vi "Scan Barcode enqueue.vi"(5 "Enum Selection":T2, 6 "Enqueue N":T1[](array[typedef]), 7 "Error In":errorcluster, 9 "Enqueue":T1, 10 "queue in":refnum<queue>) -> (0 "error out":errorcluster, 2 "D-enqueue":T1, 3 "queue Out":refnum<queue>)   [LabVIEW 2015]
uses:
  Test selectionSB.ctl
  Test seqSB.ctl
panel:
  out "Denueue N":T1[](array[typedef])
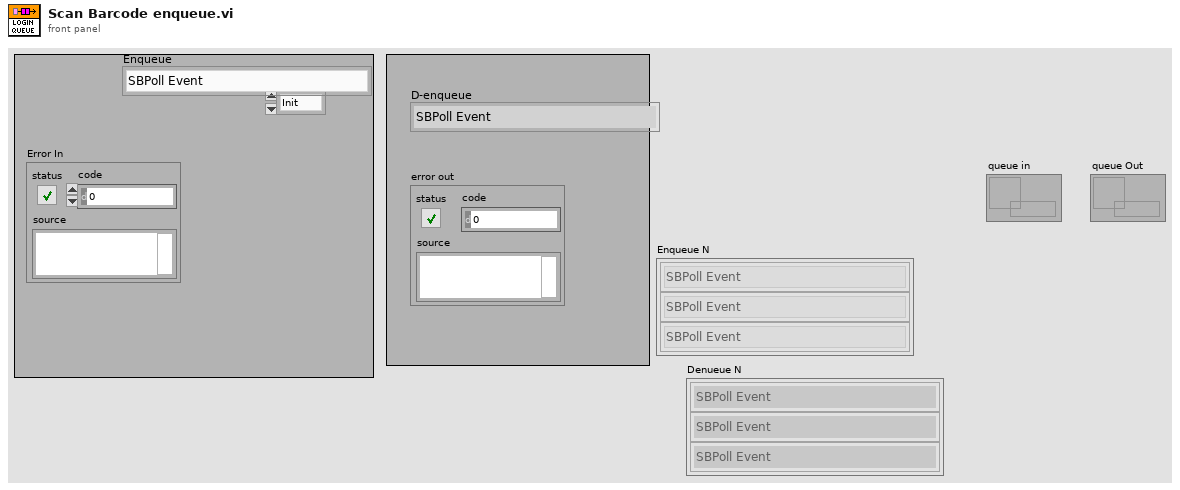
[diagram p1: front panel]
types:
  T1 = typedef "Test seqSB.ctl" = enum16{"SBPoll Event", "SBinitialize", "SB Comport Check1", "SB Comport Check2", "SB Comport Check3", "SB Comport Check4", "SB Exit"}
  T2 = typedef "Test selectionSB.ctl" = enum16{"Init", "Enqueue ", "Enqueue N", "Enqueue in stack", "Enqueue in stack N", "Dequeue", "Dequeue N", "Flush", "Release Queue"}
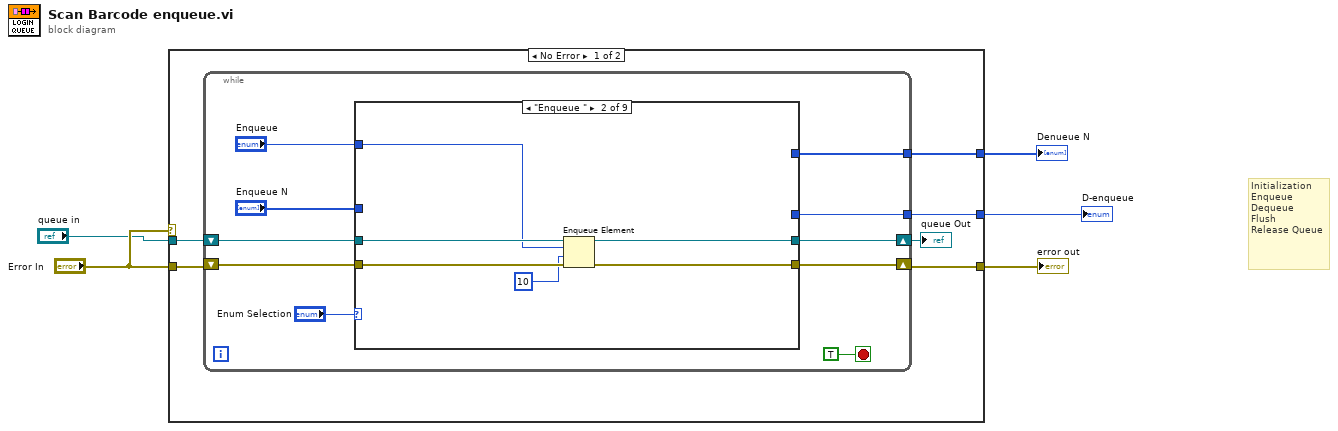
[diagram p0: block diagram]
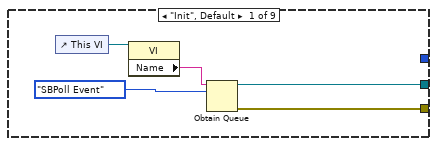
[diagram p2: hidden frame]
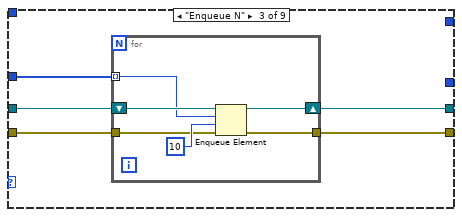
[diagram p3: hidden frame]
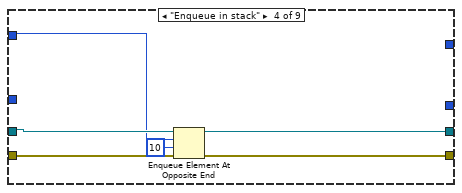
[diagram p4: hidden frame]
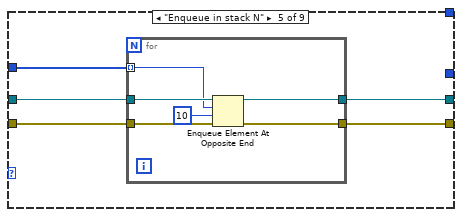
[diagram p5: hidden frame]
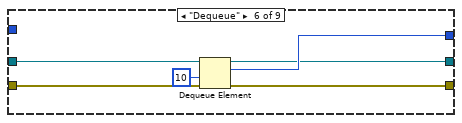
[diagram p6: hidden frame]
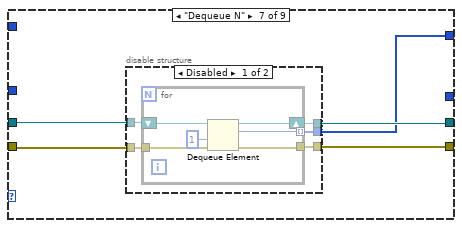
[diagram p7: hidden frame]
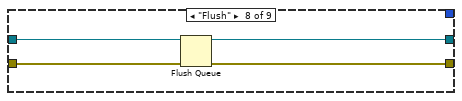
[diagram p9: hidden frame]
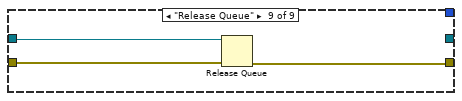
[diagram p10: hidden frame]
diagram:
  # "Initialization\nEnqueue\nDequeue\nFlush\nRelease Queue"
  n1 = case shown="No Error" "Error In" {
    tunnel: [w11 _] -> w5
    tunnel: [w10 _] -> w3
    tunnel: "Error In" -> [w9 _]
    tunnel: [w8 _] -> w2
    tunnel: "queue in" -> [w7 _]
    frame No Error {
      n2 = while {
        shift-right: [w20] -> w6
        shift-left: w7 -> [w18]
        shift-right: [w21] -> w11
        shift-left: w9 -> [w17]
        tunnel: [w15] -> w10
        tunnel: [w12] -> w8
        stop <- TRUE stop-if-true
        n3 = case shown="\"Enqueue \"" "Enum Selection" {
          tunnel: [w26 w31 w36 w48 w52 w63 w71 w84 _] -> w20
          tunnel: [w25 w30 w33 w44 w51 w62 w70 w83 w87] -> w21
          tunnel: w18 -> [_ w32 w37 w49 w54 w66 w68 w86 w89]
          tunnel: w17 -> [_ w29 w34 w47 w53 w65 w69 w85 w88]
          tunnel: [_ _ _ _ _ w64 _ _ _] -> w15
          tunnel: "Enqueue N" -> [_ _ w35 _ w50 _ _ _ _]
          tunnel: "Enqueue" -> [_ w27 _ w45 _ _ _ _ _]
          tunnel: [_ _ _ _ _ _ w67 _ _] -> w12
          frame "Init", Default {
            n4 = control-ref of="This VI"() -> (w23:refnum<vi>)
            n5 = property class="VI"(reference=w23) -> ("Name"=w24:string)  [unwired: 1 in, 2 out]
            n6 = Obtain Queue(name (unnamed)=w24, element data type=Test_seqSB."SBPoll Event" ("Enqueue")) -> (queue out=w26:refnum<queue>, error out=w25:errorcluster)  [unwired: 3 in, 1 out]
          }
          frame "Enqueue " {
            n7 = Enqueue Element(queue=w32, element=w27, timeout in ms (-1)=10, error in (no error)=w29) -> (queue out=w31:refnum<queue>, error out=w30:errorcluster)  [unwired: 1 out]
          }
          frame "Enqueue N" {
            n8 = for {
              shift-right: [w41] -> w36
              shift-left: w37 -> [w42]
              tunnel: w35 -> [w40] mode=indexing
              tunnel: w34 -> [w39]
              tunnel: [w38] -> w33
              n9 = Enqueue Element(queue=w42, element=w40, timeout in ms (-1)=10, error in (no error)=w39) -> (queue out=w41:refnum<queue>, error out=w38:errorcluster)  [unwired: 1 out]
            }
          }
          frame "Enqueue in stack" {
            n10 = Enqueue Element At Opposite End(queue=w49, element=w45, timeout in ms (-1)=10, error in (no error)=w47) -> (queue out=w48:refnum<queue>, error out=w44:errorcluster)  [unwired: 1 out]
          }
          frame "Enqueue in stack N" {
            n11 = for {
              tunnel: w54 -> [w60]
              tunnel: w53 -> [w59]
              tunnel: [w58] -> w52
              tunnel: [w57] -> w51
              tunnel: w50 -> [w55] mode=indexing
              n12 = Enqueue Element At Opposite End(queue=w60, element=w55, timeout in ms (-1)=10, error in (no error)=w59) -> (queue out=w58:refnum<queue>, error out=w57:errorcluster)  [unwired: 1 out]
            }
          }
          frame "Dequeue" {
            n13 = Dequeue Element(queue=w66, timeout in ms (-1)=10, error in (no error)=w65) -> (queue out=w63:refnum<queue>, element=w64:T1, error out=w62:errorcluster)  [unwired: 1 out]
          }
          frame "Dequeue N" {
            n14 = disable-structure shown="Disabled" {
              disable-tunnel: [w76 _] -> w71
              disable-tunnel: [w75 _] -> w70
              disable-tunnel: w69 -> [w74 _]
              disable-tunnel: w68 -> [w73 _]
              disable-tunnel: [w72 _] -> w67
              frame Disabled {
                n15 = for {
                  tunnel: [w80] -> w75
                  tunnel: w74 -> [w79]
                  shift-right: [w81] -> w76
                  shift-left: w73 -> [w78]
                  tunnel: [w77] -> w72 mode=indexing
                  n16 = Dequeue Element(queue=w78, timeout in ms (-1)=1, error in (no error)=w79) -> (queue out=w81:refnum<queue>, element=w77:T1, error out=w80:errorcluster)  [unwired: 1 out]
                }
              }
              frame Enabled {
              }
            }
          }
          frame "Flush" {
            n17 = Flush Queue(queue=w86, error in (no error)=w85) -> (queue out=w84:refnum<queue>, error out=w83:errorcluster)  [unwired: 1 out]
          }
          frame "Release Queue" {
            n18 = Release Queue(queue=w89, error in (no error)=w88) -> (error out=w87:errorcluster)  [unwired: 1 in, 2 out]
          }
        }
      }
      "queue Out" <- w6
    }
    frame Error {
    }
  }
  "error out" <- w5
  "D-enqueue" <- w3
  "Denueue N" <- w2
